vi "consigna.vi"(11 "Dial":dbl(knob) scale=0.0..6000.0) -> (3 "String":string)   [LabVIEW 2023]
panel:
  in  "stop":bool
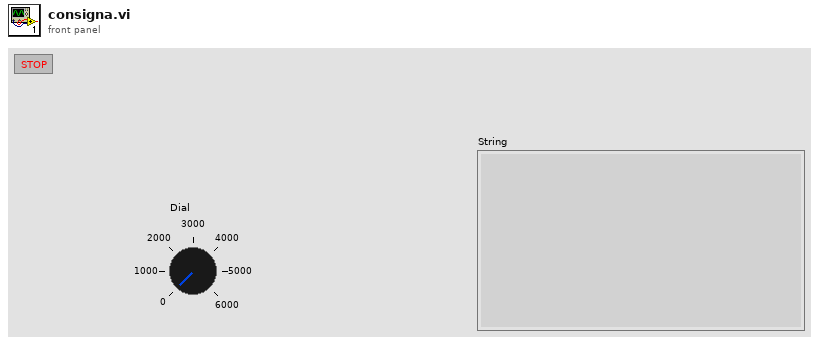
[diagram p1: front panel]
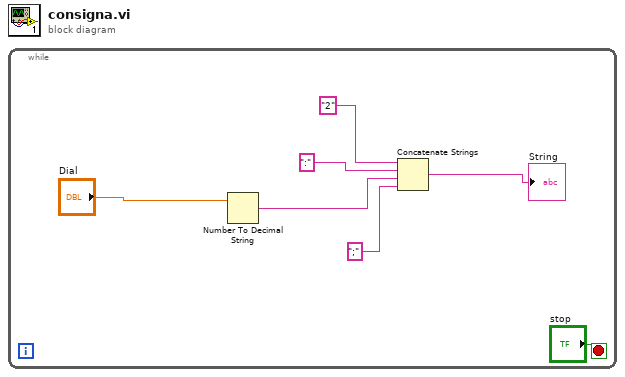
[diagram p0: block diagram]
diagram:
  n1 = while {
    stop <- "stop" stop-if-true
    n2 = Number To Decimal String(number="Dial") -> (decimal integer string=w7:string)  [unwired: 1 in]
    n3 = Concatenate Strings("2" ("string"), ":" ("string"), w7, ";" ("string")) -> (→"String":string)
  }
